vi "GetSubVIStartPoint.vi"(1 "Subroutine (runs prgm if unwired)":string) -> (0 "String":string)   [LabVIEW 2014]
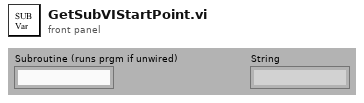
[diagram p1: front panel]
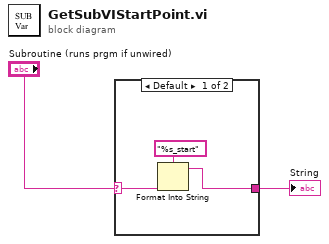
[diagram p0: block diagram]
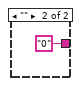
[diagram p2: hidden frame]
diagram:
  n1 = case shown="Default" "Subroutine (runs prgm if unwired)" {
    selector: "Subroutine (runs prgm if unwired)" -> [w5 _]
    tunnel: [w3 "0"] -> w2
    frame Default {
      n2 = Format Into String(format string="%s_start" ("String"), w5) -> (resulting string=w3:string)  [unwired: 2 in, 1 out]
    }
    frame "" {
    }
  }
  "String" <- w2
